vi "EnqueueMessage.vi"(6 "Priority?":bool, 8 "error in (no error)":errorcluster, 9 "Data":variant, 10 "Command":string, 11 "Queue in":refnum<queue>) -> (0 "error out":errorcluster, 3 "Queue out":refnum<queue>)   [LabVIEW 2013, in "Message Queue.lvlib"]
uses:
  ctl_MessageQueue.ctl
  Message Queue.lvlib
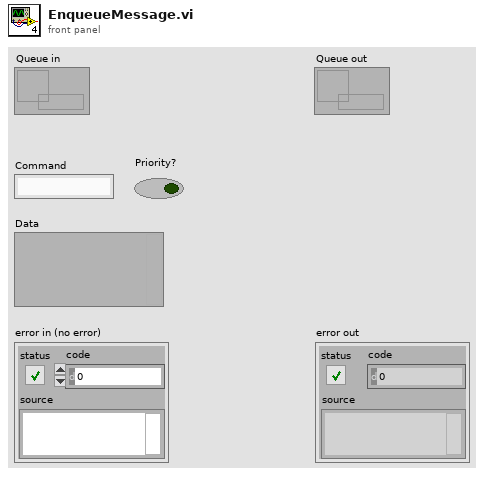
[diagram p1: front panel]
types:
  T1 = typedef "Message Queue.lvlib/ctl_MessageQueue.ctl" = cluster{"Command":string, "Data":variant}
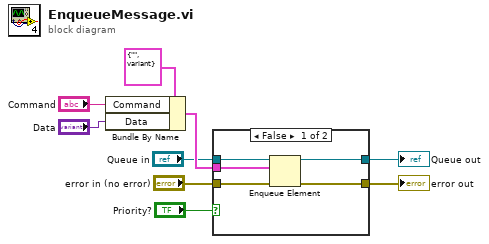
[diagram p0: block diagram]
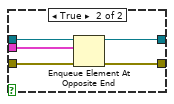
[diagram p2: hidden frame]
diagram:
  n1 = Bundle By Name(cluster=T1 {"Command"="", "Data"=variant}, "Command"="Command", "Data"="Data") -> (w7:T1)
  n2 = case shown="False" "Priority?" {
    tunnel: w7 -> [w14 w15]
    tunnel: "Queue in" -> [w13 w18]
    tunnel: [w12 w19] -> w4
    tunnel: "error in (no error)" -> [w11 w16]
    tunnel: [w10 w17] -> w2
    frame False {
      n3 = Enqueue Element(queue=w13, element=w14, error in (no error)=w11) -> (queue out=w12:refnum<queue>, error out=w10:errorcluster)  [unwired: 1 in, 1 out]
    }
    frame True {
      n4 = Enqueue Element At Opposite End(queue=w18, element=w15, error in (no error)=w16) -> (queue out=w19:refnum<queue>, error out=w17:errorcluster)  [unwired: 1 in, 1 out]
    }
  }
  "Queue out" <- w4
  "error out" <- w2
